vi "intervalo2.vi"(9 "incremento":dbl, 10 "fin":dbl, 11 "inicio":dbl) -> (2 "Array":dbl[](array[numeric]))   [LabVIEW 2016]
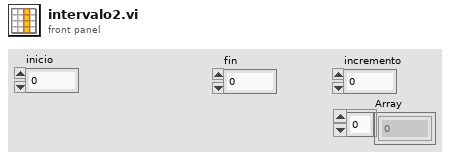
[diagram p1: front panel]
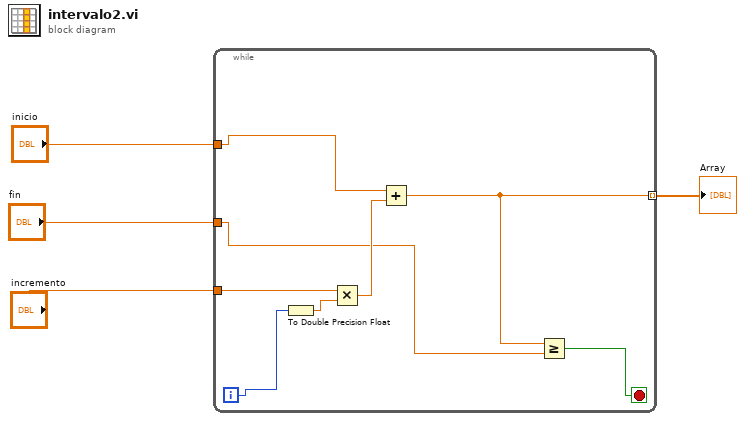
[diagram p0: block diagram]
diagram:
  n1 = while {
    tunnel: "inicio" -> [w12]
    tunnel: "fin" -> [w5]
    tunnel: "incremento" -> [w11]
    tunnel: [w6] -> w1 mode=indexing
    i -> [w9]
    stop <- w7 stop-if-true
    n2 = To Double Precision Float(number=w9) -> (double precision float=w10:dbl)
    n3 = Multiply(x=w11, y=w10) -> (x*y=w8:dbl)
    n4 = Add(x=w12, y=w8) -> (x+y=w6:dbl)
    n5 = Greater Or Equal?(x=w6, y=w5) -> (x >= y?=w7:bool)
  }
  "Array" <- w1
